vi "Create_Job_In_TreeControl.vi"(8 "error in (no error)":errorcluster, 10 "Left Cell String":string="JOB", 11 "TreeControl in":refnum<vi>) -> (0 "error out":errorcluster, 2 "Edit Tree Items:Add Item":string, 3 "TreeControl out":refnum<vi>)   [LabVIEW 2021]
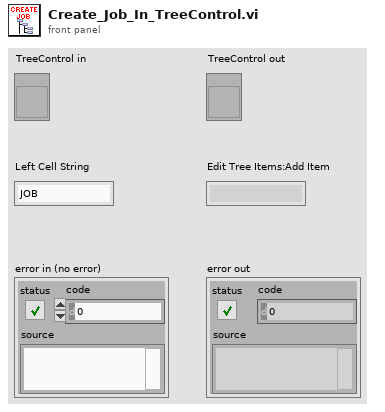
[diagram p1: front panel]
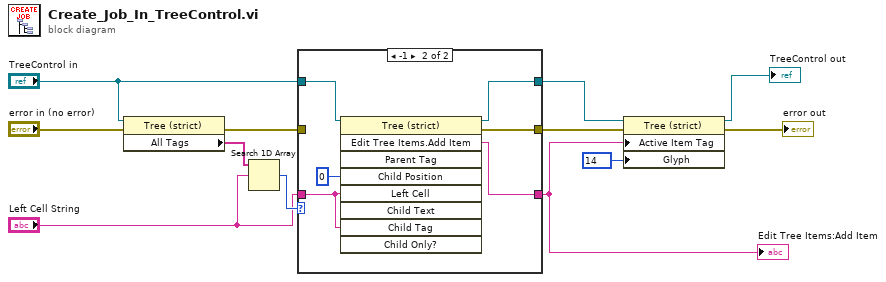
[diagram p0: block diagram]
diagram:
  n1 = property on="Property Node" class="Tree (strict)"(reference="TreeControl in", error in="error in (no error)") -> (error out=w12:errorcluster, "All Tags"=w9:string[])  [unwired: 1 out]
  n2 = Search 1D Array(1D array=w9, element="Left Cell String") -> (index of element=w11:i32)  [unwired: 1 in]
  n3 = case shown="-1" w11 {
    tunnel: [w14 w20] -> w5
    tunnel: [w15 w19] -> w3
    tunnel: "Left Cell String" -> [w15 w18]
    tunnel: w12 -> [w14 _]
    tunnel: "TreeControl in" -> [w13 w17]
    tunnel: [w13 w16] -> w6
    frame 0, Default {
    }
    frame -1 {
      n4 = invoke on="Invoke Node" class="Tree (strict)" method="Edit Tree Items.Add Item"(reference=w17, "Child Position"=0, "Left Cell"=w18, "Child Tag"=w18) -> (reference out=w16:refnum<vi>, error out=w20:errorcluster, "Edit Tree Items:Add Item"=w19:string)  [unwired: 5 in, 6 out]
    }
  }
  "Edit Tree Items:Add Item" <- w3
  n5 = property class="Tree (strict)"(reference=w6, error in=w5, "Active Item Tag"=w3, "Glyph"=14) -> (reference out=→"TreeControl out":refnum<vi>, error out=→"error out":errorcluster)
